vi "execute.vi"(8 "error in (no error)":errorcluster, 9 "ParameterString":string, 10 "ObjectCluster":T1, 11 "Command in":refnum<class "Command.lvclass">) -> (0 "error out":errorcluster, 2 "ObjectCluster Out":T1, 3 "Command out":refnum<class "Command.lvclass">)   [LabVIEW 2013, in "Command.lvclass"]
uses:
  Command.lvclass
  ObjectCluster.ctl
  AirCondition.lvclass/AirCondition.lvclass
  RoomLight.lvclass/RoomLight.lvclass
  OutDoorLight.lvclass/OutDoorLight.lvclass
  Television.lvclass/Television.lvclass
  Stereo.lvclass/Stereo.lvclass
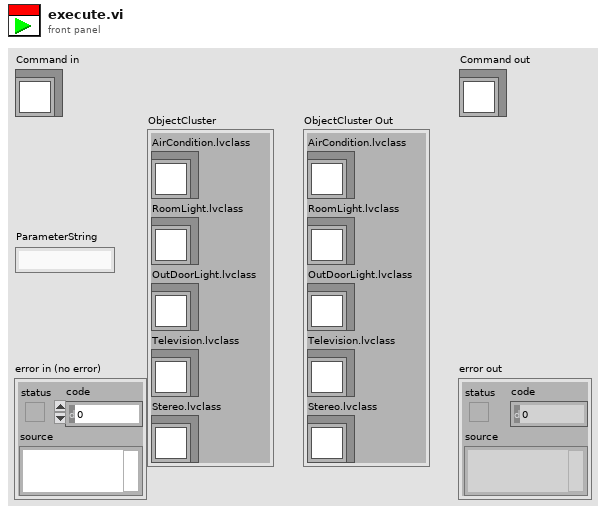
[diagram p1: front panel]
types:
  T1 = typedef "Command.lvclass/ObjectCluster.ctl" = cluster{"AirCondition.lvclass":refnum<class "AirCondition.lvclass">, "RoomLight.lvclass":refnum<class "RoomLight.lvclass">, "OutDoorLight.lvclass":refnum<class "OutDoorLight.lvclass">, "Television.lvclass":refnum<class "Television.lvclass">, "Stereo.lvclass":refnum<class "Stereo.lvclass">}
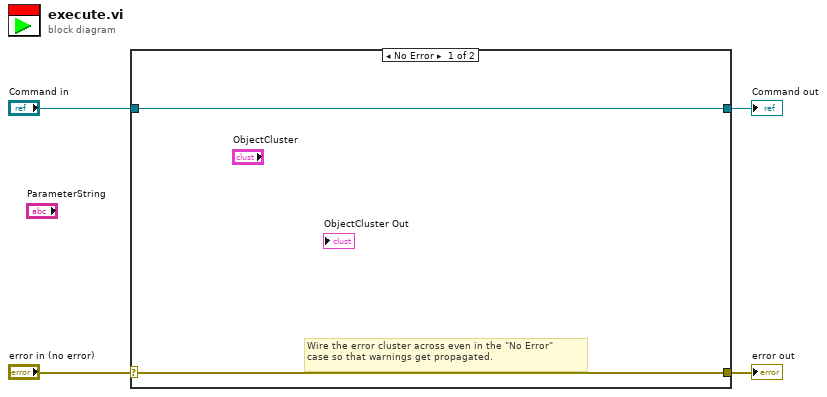
[diagram p0: block diagram]
diagram:
  n1 = case shown="No Error" "error in (no error)" {
    selector: "error in (no error)" -> [w5 w8]
    tunnel: [w5 w8] -> w3
    tunnel: [w6 w7] -> w1
    tunnel: "Command in" -> [w6 w7]
    frame No Error {
      # "Wire the error cluster across even in the \"No Error\"\ncase so that warnings get propagated."
    }
    frame Error {
    }
  }
  "error out" <- w3
  "Command out" <- w1
